vi "autoscroll.vi"(8 "error in (no error)":errorcluster, 10 "Table in":refnum<vi>, 11 "State":T1={"logTable"=refnum, "max items"=500, "displaydata"=[], "data"=[], "Auto Scroll"=TRUE, "current item"=500, "col headers"=[], "Add to Top"=TRUE, "Auto resize"=TRUE, "col size"=[], "filters"=[], "color cells"=[]}) -> (0 "error out":errorcluster, 1 "Number of Rows":i32, 2 "Table out":refnum<vi>, 3 "State (dup)":T1={"logTable"=refnum, "max items"=500, "displaydata"=[], "data"=[], "Auto Scroll"=TRUE, "current item"=500, "col headers"=[], "Add to Top"=TRUE, "Auto resize"=TRUE, "col size"=[], "filters"=[], "color cells"=[]})   [LabVIEW 2013, in "UI-DisplayTable(dev).xctl"]
uses:
  UI-DisplayTable(dev).xctl
  State.ctl
  DEF-Filter.ctl
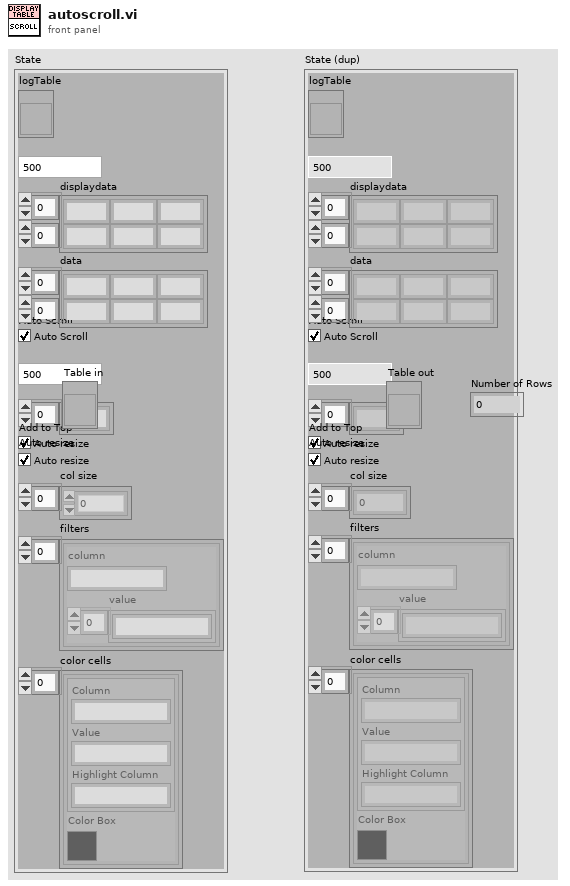
[diagram p1: front panel]
types:
  T1 = typedef "UI-DisplayTable(dev).xctl/State.ctl" = cluster{"logTable":refnum<vi>, "max items":i32, "displaydata":string[][], "data":string[][], "Auto Scroll":bool, "current item":i32, "col headers":string[], "Add to Top":bool, "Auto resize":bool, "col size":i32[], "filters":T2[], "color cells":cluster{"color cell":cluster{"Column":string, "Value":string, "Highlight Column":string}, "Color Box":u32}[]}
  T2 = typedef "UI-DisplayTable(dev).xctl/DEF-Filter.ctl" = cluster{"column":string, "value":string[]}
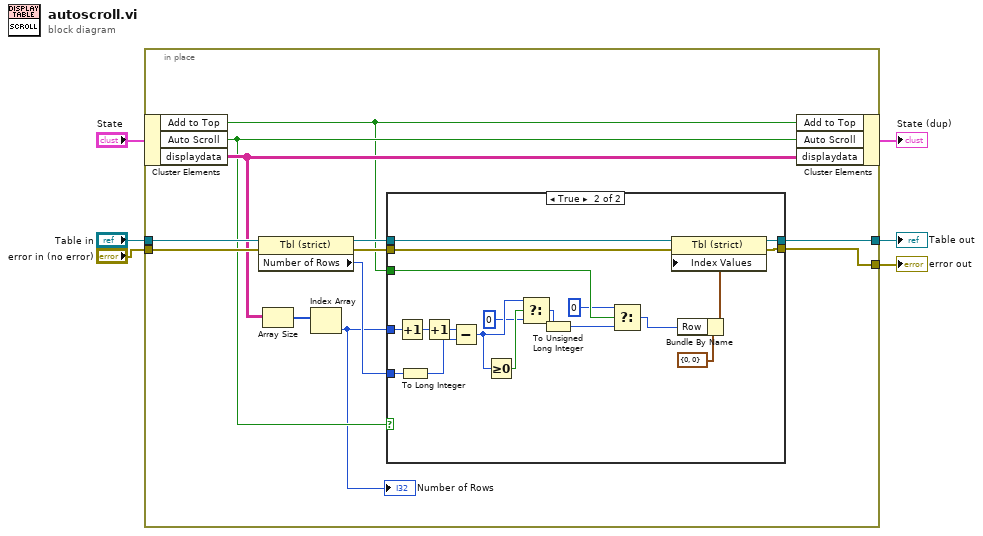
[diagram p0: block diagram]
diagram:
  n1 = in-place {
    in-place-border: "Table in" -> [w14]
    in-place-border: "error in (no error)" -> [w13]
    in-place-border: [w12] -> w2
    in-place-border: [w11] -> w1
    n2 = in-place-cluster #1("State") -> ("Add to Top"=w8:bool, "Auto Scroll"=w9:bool, "displaydata"=w10:string[][])
    n3 = property on="Property Node" class="Tbl (strict)"(reference=w14, error in=w13) -> (reference out=w17:refnum<vi>, error out=w18:errorcluster, "Number of Rows"=w16:u32)
    n4 = Array Size(array=w10) -> (size(s)=w15:i32[])
    n5 = Index Array(array=w15) -> (element=w7:i32)  [unwired: 1 in]
    "Number of Rows" <- w7
    n6 = case shown="True" w9 {
      tunnel: w18 -> [w20 w39]
      tunnel: w17 -> [w19 w35]
      tunnel: [w20 w34] -> w11
      tunnel: w16 -> [_ w33]
      tunnel: w7 -> [_ w32]
      tunnel: [w19 w25] -> w12
      tunnel: w8 -> [_ w24]
      frame False {
      }
      frame True {
        n7 = Increment(x=w32) -> (x+1=w27:i32)
        n8 = To Long Integer(number=w33) -> (32bit integer=w26:i32)
        n9 = Increment(x=w27) -> (x+1=w28:i32)
        n10 = Subtract(x=w28, y=w26) -> (x-y=w30:i32)
        n11 = Greater Or Equal To 0?(x=w30) -> (x >= 0?=w31:bool)
        n12 = Select(t=w30, s=w31, f=0) -> (s? t:f=w36:i32)
        n13 = To Unsigned Long Integer(number=w36) -> (unsigned 32bit integer=w23:u32)
        n14 = Select(t=u32 0, s=w24, f=w23) -> (s? t:f=w22:u32)
        n15 = Bundle By Name(cluster=cluster{"Row":u32, "Column":u32} {"Row"=0, "Column"=0} ("Index Values"), "Row"=w22) -> (w37:cluster{"Row":u32, "Column":u32})
        n16 = property on="Property Node" class="Tbl (strict)"(reference=w35, error in=w39, "Index Values"=w37) -> (reference out=w25:refnum<vi>, error out=w34:errorcluster)
      }
    }
    n17 = in-place-cluster #1("Add to Top"=w8, "Auto Scroll"=w9, "displaydata"=w10) -> (→"State (dup)":T1)
  }
  "error out" <- w1
  "Table out" <- w2
